vi "execution ui.vi"() -> ()   [LabVIEW 2013, in "VI modification collection.lvclass"]
uses:
  VI modification collection.lvclass
  <vilib>/CEF_TreeControl/Node/NodeRef.ctl
  <vilib>/CEF_TreeControl/Node/NISE_CEF_Node.lvclass
  <vilib>/NI/AMC/Message Queue.ctl
  <vilib>/NI/AMC/Message.ctl
  <vilib>/NI/Tools/Keyed Array/KeyedArray.ctl
  <vilib>/CEF_TreeControl/Node/UserEventRef.ctl
  <vilib>/CEF_TreeControl/Controls/EventCluster.ctl
  VI modification collection.lvclass/VI modification collection.ctl
  <vilib>/NI/Tools/Keyed Array/Tools_KeyedArray.lvlib
  <vilib>/NI/AMC/AMC.lvlib
  <vilib>/CEF_TreeControl/NISE_CEF_TreeControl.lvlib
panel:
  in  "Remove path":bool
  in  "add search":bool
  in  "Paths":i32(listbox)
  in  "run":bool
  in  "user event":T1
  in  "main queue":T2
  in  "node ref":T3
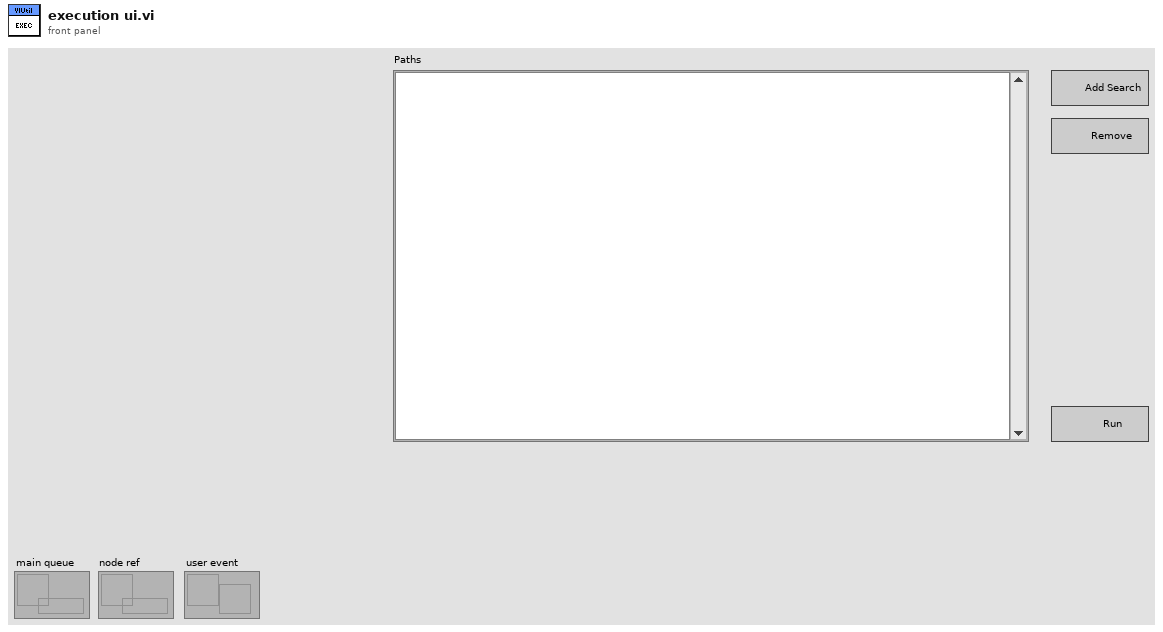
[diagram p1: front panel]
types:
  T1 = typedef "NISE_CEF_Node.lvclass/UserEventRef.ctl" = refnum<user-event>
  T2 = typedef "AMC.lvlib/Message Queue.ctl" = refnum<queue>
  T3 = typedef "NISE_CEF_Node.lvclass/NodeRef.ctl" = refnum<data-value>
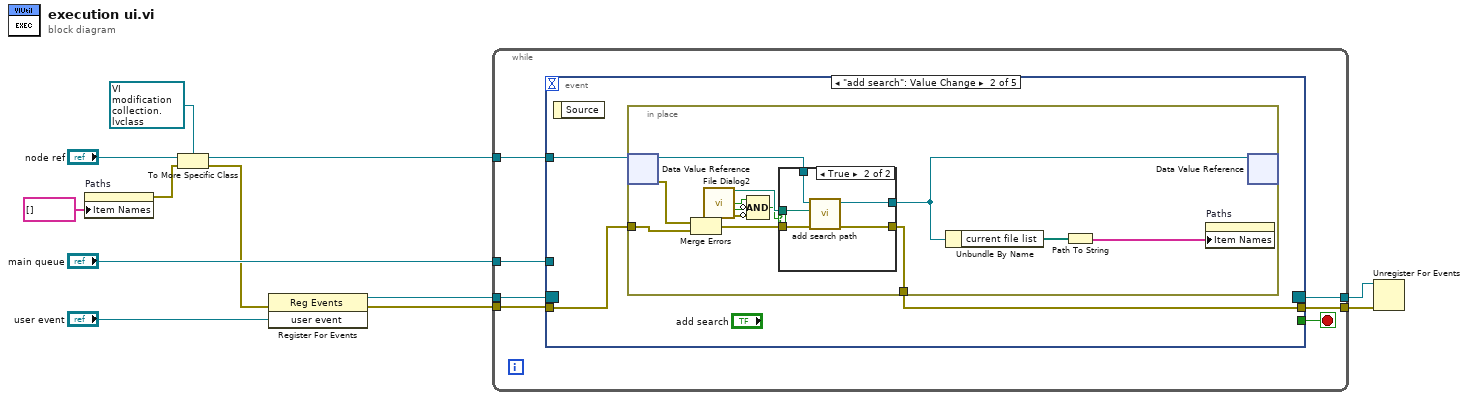
[diagram p0: block diagram]
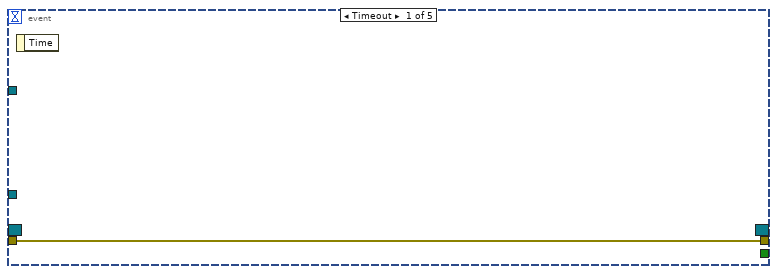
[diagram p2: hidden frame]
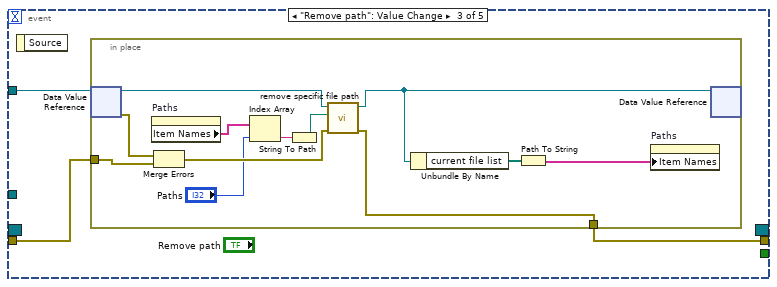
[diagram p4: hidden frame]
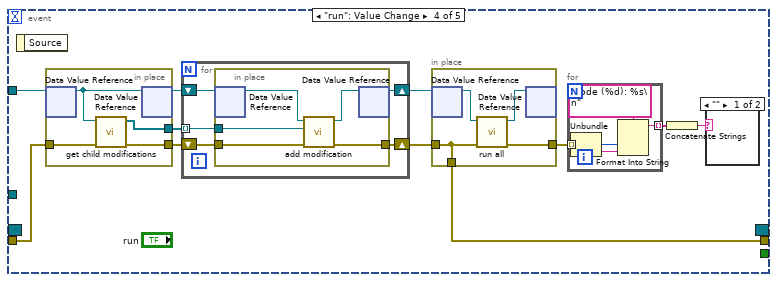
[diagram p5: hidden frame]
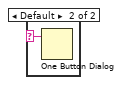
[diagram p6: hidden frame]
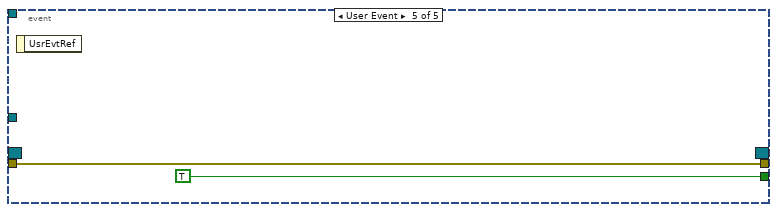
[diagram p7: hidden frame]
diagram:
  n1 = property on="Paths" class="LstBox (strict)"("Item Names"=string[] []) -> (error out=w2:errorcluster)  [unwired: 2 in, 1 out]
  n2 = To More Specific Class(target class=refnum<data-value> refnum ("node ref 2"), reference="node ref", error in=w2) -> (specific class reference=w5:refnum<data-value>, error out=w3:errorcluster)
  n3 = register-events(error in=w3, "user event") -> (reference out=w9:refnum<event-registration>, error out=w6:errorcluster)  [unwired: 1 in]
  n4 = while {
    tunnel: w5 -> [w19]
    tunnel: "main queue" -> [w18]
    tunnel: w9 -> [w17]
    tunnel: [w16] -> w8
    tunnel: [w14] -> w7
    tunnel: w6 -> [w13]
    stop <- w15 stop-if-true
    n5 = event shown="[1] \"add search\": Value Change" {
      selector: w17 -> [_ _ _ _ _]
      dyn-events: [_ _ _ _ _] -> w16
      timeout: _ -> [_ _ _ _ _]
      tunnel: w19 -> [_ w23 w46 w69 _]
      tunnel: w18 -> [_ _ _ _ _]
      tunnel: [_ _ _ _ TRUE] -> w15
      tunnel: [w20 w21 w44 w62 w94] -> w14
      tunnel: w13 -> [w20 w22 w45 w63 w94]
      event Timeout {
        n6 = event-data() -> ()  [unwired: 1 in, 1 out]
      }
      event "add search": Value Change {
        n7 = event-data() -> ()  [unwired: 1 in, 1 out]
        n8 = in-place {
          in-place-border: w22 -> [w31]
          in-place-border: [w27] -> w21
          n9 = in-place-dvr #1(w23) -> (w28:refnum<class "VI modification collection.lvclass">, w29:errorcluster)
          n10 = Merge Errors(w29, w31) -> (w30:errorcluster)
          n11 = call "File Dialog2"() -> ("selected path"=w33:path, "exists"=w34:bool, "cancelled"=w35:bool, "error out"=w36:errorcluster)  [unwired: 12 in]
          n12 = Compound Arithmetic op=AND(w34, invert w35, invert w36) -> (w32:bool)
          n13 = case shown="True" w32 {
            tunnel: w30 -> [w37 w43]
            tunnel: [w37 w42] -> w27
            tunnel: w28 -> [w38 w41]
            tunnel: [w38 w40] -> w25
            tunnel: w33 -> [_ w39]
            frame False {
            }
            frame True {
              n14 = call "add search path.vi"("error in"=w43, "Path"=w39, "vi modification tool in"=w41) -> ("error out"=w42:errorcluster, "vi modification tool out"=w40:refnum<class "VI modification collection.lvclass">)  [unwired: 7 in]
            }
          }
          n15 = Unbundle By Name(w25) -> ("current file list"=w24:path[])
          n16 = Path To String(path=w24) -> (string=w26:string[])
          n17 = property on="Paths" class="LstBox (strict)"("Item Names"=w26) -> ()  [unwired: 2 in, 2 out]
          n18 = in-place-dvr #1(w25) -> ()  [unwired: 2 out]
        }
      }
      event "Remove path": Value Change {
        n19 = event-data() -> ()  [unwired: 1 in, 1 out]
        n20 = in-place {
          in-place-border: w45 -> [w58]
          in-place-border: [w51] -> w44
          n21 = in-place-dvr #2(w46) -> (w53:refnum<class "VI modification collection.lvclass">, w57:errorcluster)
          n22 = property on="Paths" class="LstBox (strict)"() -> ("Item Names"=w49:string[])  [unwired: 2 in, 2 out]
          n23 = Merge Errors(w57, w58) -> (w52:errorcluster)
          n24 = Index Array(array=w49, index="Paths") -> (element=w50:string)
          n25 = String To Path(string=w50) -> (path=w48:path)
          n26 = call "remove specific file path.vi"("error in"=w52, "Path"=w48, "VI modification collection in"=w53) -> ("error out"=w51:errorcluster, "VI modification collection out"=w54:refnum<class "VI modification collection.lvclass">)  [unwired: 7 in]
          n27 = Unbundle By Name(w54) -> ("current file list"=w55:path[])
          n28 = Path To String(path=w55) -> (string=w56:string[])
          n29 = property on="Paths" class="LstBox (strict)"("Item Names"=w56) -> ()  [unwired: 2 in, 2 out]
          n30 = in-place-dvr #2(w54) -> ()  [unwired: 2 out]
        }
      }
      event "run": Value Change {
        n31 = event-data() -> ()  [unwired: 1 in, 1 out]
        n32 = in-place {
          in-place-border: w63 -> [w83]
          in-place-border: [w82] -> w68
          in-place-border: [w80] -> w66
          n33 = in-place-dvr #3(w69) -> (w81:refnum<class "VI modification collection.lvclass">)  [unwired: 1 out]
          n34 = call "get child modifications.vi"("error in"=w83, "VI modification collection in"=w81) -> ("error out"=w82:errorcluster, "modifications"=w80:refnum<class "VI modification.lvclass">[])  [unwired: 8 in]
          n35 = in-place-dvr #3(w81) -> (w67:refnum<data-value>)  [unwired: 1 out]
        }
        n36 = for {
          shift-right: [w87] -> w65
          shift-left: w68 -> [w88]
          tunnel: w66 -> [w84] mode=indexing
          shift-right: [w85] -> w64
          shift-left: w67 -> [w86]
          n37 = in-place {
            in-place-border: w88 -> [w93]
            in-place-border: [w92] -> w87
            in-place-border: w84 -> [w89]
            n38 = in-place-dvr #4(w86) -> (w91:refnum<class "VI modification collection.lvclass">)  [unwired: 1 out]
            n39 = call "add modification.vi"("error in"=w93, "VI modification"=w89, "vi modification tool in"=w91) -> ("error out"=w92:errorcluster, "vi modification tool out"=w90:refnum<class "VI modification collection.lvclass">)  [unwired: 7 in]
            n40 = in-place-dvr #4(w90) -> (w85:refnum<data-value>)  [unwired: 1 out]
          }
        }
        n41 = in-place {
          in-place-border: w65 -> [w78]
          in-place-border: [w79] -> w61
          in-place-border: [w78] -> w62
          n42 = in-place-dvr #5(w64) -> (w77:refnum<class "VI modification collection.lvclass">)  [unwired: 1 out]
          n43 = call "run all.vi"("error in"=w78, "vi modification tool in"=w77) -> ("error report"=w79:errorcluster[], "vi modification tool out"=w76:refnum<class "VI modification collection.lvclass">)  [unwired: 8 in]
          n44 = in-place-dvr #5(w76) -> ()  [unwired: 2 out]
        }
        n45 = for {
          tunnel: w61 -> [w75] mode=indexing
          tunnel: [w71] -> w60 mode=indexing
          n46 = Unbundle(w75) -> ("code"=w74:i32, "source"=w73:string)  [unwired: 1 out]
          n47 = Format Into String(format string="code (%d): %s\n", w74, w73) -> (resulting string=w71:string)  [unwired: 2 in, 1 out]
        }
        n48 = Concatenate Strings(w60) -> (w59:string)
        n49 = case shown="\"\"" w59 {
          selector: w59 -> [_ w70]
          frame "" {
          }
          frame Default {
            n50 = One Button Dialog(message=w70) -> ()  [unwired: 1 in, 1 out]
          }
        }
      }
      event User Event {
        n51 = event-data() -> ()  [unwired: 1 in, 1 out]
      }
    }
  }
  n52 = Unregister For Events(event registration refnum=w8, error in=w7) -> ()  [unwired: 1 out]
